vi "SPI Initialise.vi"(8 "error in (no error)":errorcluster, 11 "LINX SPI in":refnum<class "LINX SPI.lvclass">) -> (0 "error out":errorcluster, 3 "LINX SPI out":refnum<class "LINX SPI.lvclass">)   [LabVIEW 2020, in "LINX SPI.lvclass"]
uses:
  LINX SPI.lvclass
  LINX SPI.lvclass/LINX SPI.ctl
  Read LINX Resource.vi
  Read SPI Channel (0).vi
  Read SPI Configuration.vi
  Write LINX Resource.vi
  <vilib>/MakerHub/LINX/LMH-LINX.lvlib
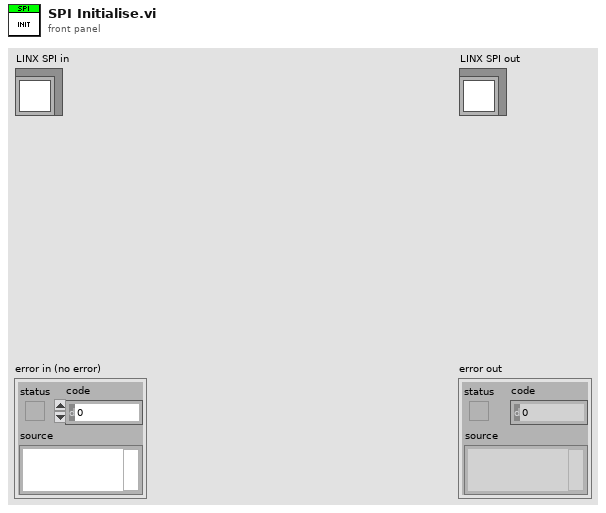
[diagram p1: front panel]
types:
  T1 = typedef "LMH-LINX.lvlib/LINX Ref.ctl" = cluster{"IO":T2, "Interface":T3, "LINX Device Config":T4}
  T2 = typedef "LMH-LINX.lvlib/Platform.ctl" = enum16{"Remote", "Local"}
  T3 = typedef "LMH-LINX.lvlib/Interface.ctl" = enum16{"Serial", "TCP"}
  T4 = typedef "LMH-LINX.lvlib/Device.lvlib/LINX Device Config.ctl" = cluster{"Interface":T3, "COM Port":refnum<visa-resource-name>, "TCP Configuration":T5, "Device Family":u8, "Device ID":u8, "Device Name":string, "TCP Ref":refnum<k5>, "Channels":T6}
  T5 = typedef "LMH-LINX.lvlib/Device.lvlib/TCP Config.ctl" = cluster{"IP Address":string, "Port":u16}
  T6 = typedef "LMH-LINX.lvlib/Channels.ctl" = cluster{"DI":u8[], "DO":u8[], "AI":u8[], "AO":u8[], "PWM":u8[], "QE":u8[], "UART":u8[], "I2C 2":u8[], "SPI":u8[], "CAN":u8[], "Servo":u8[], "AI Ref (V)":dbl, "AI Resolution (Bits)":u8, "AO Ref (V)":dbl, "AO Resolution (Bits)":u8}
  T7 = typedef "LMH-LINX.lvlib/SPI Configuration.ctl" = cluster{"Clock Frequency":u32, "Bit Order":T8, "SPI Mode":T9}
  T8 = typedef "LMH-LINX.lvlib/SPI Bit Order.ctl" = enum8{"LSb First", "MSb First"}
  T9 = typedef "LMH-LINX.lvlib/SPI Mode.ctl" = enum8{"Mode 0", "Mode 1", "Mode 2", "Mode 3"}
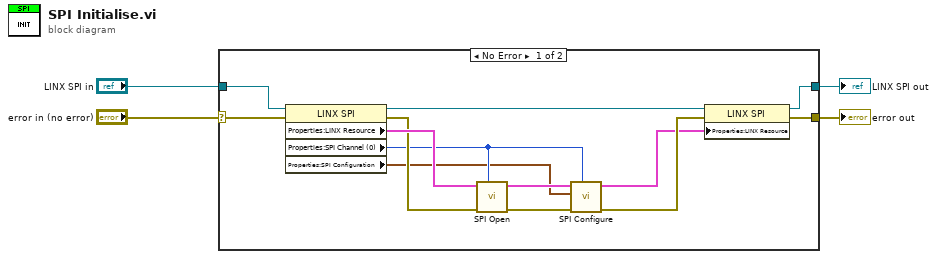
[diagram p0: block diagram]
diagram:
  n1 = case shown="No Error" "error in (no error)" {
    selector: "error in (no error)" -> [w16 w19]
    tunnel: [w9 w19] -> w3
    tunnel: [w11 w18] -> w1
    tunnel: "LINX SPI in" -> [w17 w18]
    frame No Error {
      n2 = property class="LINX SPI"(reference=w17, error in=w16) -> (reference out=w12:refnum<class "LINX SPI.lvclass">, error out=w13:errorcluster, "Properties:LINX Resource"=w15:T1, "Properties:SPI Channel (0)"=w6:u8, "Properties:SPI Configuration"=w5:T7)
      n3 = call <vilib>:"SPI Open.vi"("SPI Channel (0)"=w6, "Error In"=w13, "LINX Resource"=w15) -> ("Error Out"=w14:errorcluster, "LINX Resource"=w10:T1)  [unwired: 7 in]
      n4 = call <vilib>:"SPI Configure.vi"("SPI Channel (0)"=w6, "Error In"=w14, "SPI Configuration"=w5, "LINX Resource"=w10) -> ("Error Out"=w8:errorcluster, "LINX Resource"=w7:T1)  [unwired: 5 in, 1 out]
      n5 = property class="LINX SPI"(reference=w12, error in=w8, "Properties:LINX Resource"=w7) -> (reference out=w11:refnum<class "LINX SPI.lvclass">, error out=w9:errorcluster)
    }
    frame Error {
    }
  }
  "error out" <- w3
  "LINX SPI out" <- w1
